vi "ext_pressure_step_test.vi"() -> ()   [LabVIEW 2014]
panel:
  out "running now":bool
  out "Current step":dbl
  out "Total steps":dbl
  out "RH steps":dbl[](array[numeric])
  in  "start sequence":bool
  in  "config  steps cluster":T1 caption="Configure RH steps"
  in  "Stop Button":bool
  out "Current RH":dbl
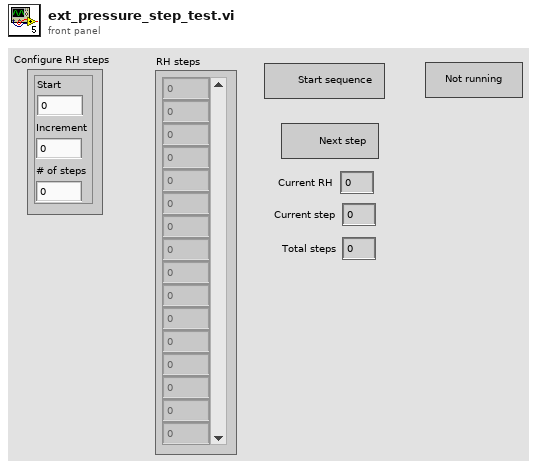
[diagram p1: front panel]
types:
  T1 = cluster{"Start":dbl, "Increment":dbl, "# of steps":i32}
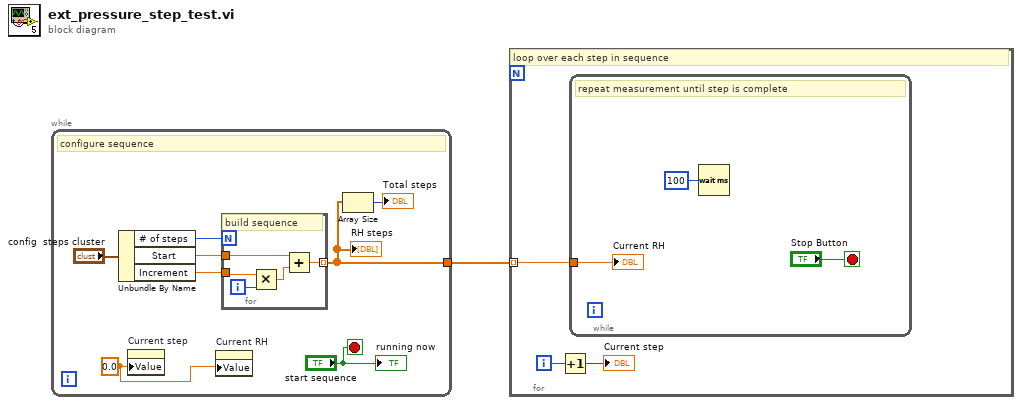
[diagram p0: block diagram]
diagram:
  n1 = while {
    tunnel: [w5] -> w1
    stop <- "start sequence" stop-if-true
    w3 = 0.0 ("Current step")
    # "configure sequence"
    n2 = Unbundle By Name("config  steps cluster") -> ("# of steps"=w8:i32, "Start"=w7:dbl, "Increment"=w6:dbl)
    n3 = property on="Current step" class="DigNum (strict)"("Value"=w3) -> ()  [unwired: 2 in, 2 out]
    n4 = property on="Current RH" class="DigNum (strict)"("Value"=w3) -> ()  [unwired: 2 in, 2 out]
    n5 = for {
      N: w8 -> [_]
      tunnel: w7 -> [w14]
      tunnel: w6 -> [w12]
      tunnel: [w10] -> w5 mode=indexing
      i -> [w13]
      # "build sequence"
      n6 = Multiply(x=w12, y=w13) -> (x*y=w11:dbl)
      n7 = Add(x=w14, y=w11) -> (x+y=w10:dbl)
    }
    "RH steps" <- w5
    n8 = Array Size(array=w5) -> (size(s)=→"Total steps":i32)
    "running now" <- "start sequence"
  }
  n9 = for {
    tunnel: w1 -> [w17] mode=indexing
    i -> [w16]
    # "loop over each step in sequence"
    n10 = Increment(x=w16) -> (x+1=→"Current step":i32)
    n11 = while {
      tunnel: w17 -> [w18]
      stop <- "Stop Button" stop-if-true
      # "repeat measurement until step is complete"
      n12 = Wait (ms)(milliseconds to wait=u32 100) -> ()  [unwired: 1 out]
      "Current RH" <- w18
    }
  }
